vi "Write AI.vi"(8 "error in (no error)":errorcluster, 10 "AI":T1, 11 "cCRDS in":refnum<class "cCRDS.lvclass">) -> (0 "error out":errorcluster, 3 "cCRDS out":refnum<class "cCRDS.lvclass">)   [LabVIEW 2012, in "cCRDS.lvclass"]
uses:
  cCRDS.lvclass
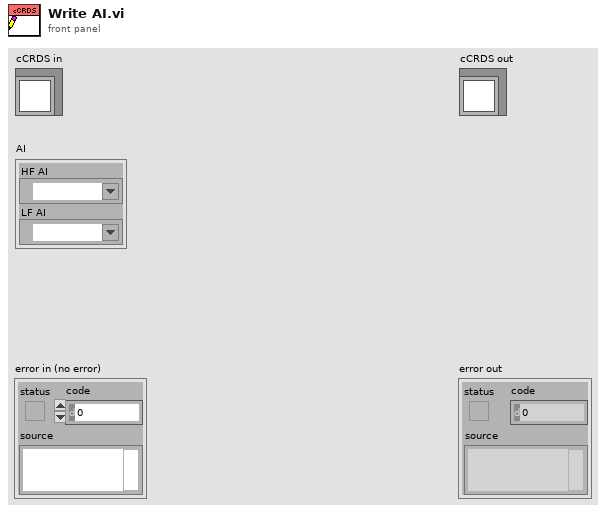
[diagram p1: front panel]
types:
  T1 = cluster{"HF AI":refnum<k21>, "LF AI":refnum<k21>}
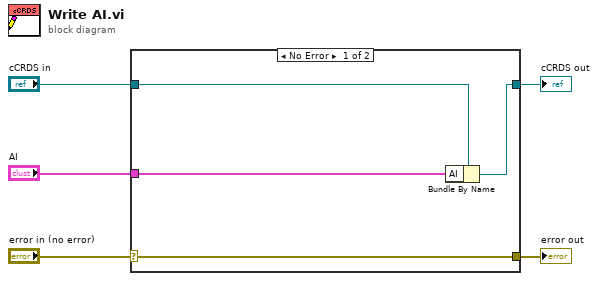
[diagram p0: block diagram]
diagram:
  n1 = case shown="No Error" "error in (no error)" {
    selector: "error in (no error)" -> [w9 w10]
    tunnel: [w9 w10] -> w4
    tunnel: [w7 w11] -> w2
    tunnel: "cCRDS in" -> [w8 w11]
    tunnel: "AI" -> [w6 _]
    frame No Error {
      n2 = Bundle By Name(cluster=w8, "AI"=w6) -> (w7:refnum<class "cCRDS.lvclass">)
    }
    frame Error {
    }
  }
  "error out" <- w4
  "cCRDS out" <- w2
